vi "DDA.vi"(8 "error in (no error)":errorcluster, 11 "Box Length X (4)":sgl=4.0) -> (0 "error out":errorcluster, 3 "SceneObject out":refnum<vi>)   [LabVIEW 2026, in "XRay CArm.lvclass"]
uses:
  XRay CArm.lvclass
  <vilib>/picture/3D Picture Control/Object/Create Object (drawable).vi
  <vilib>/picture/3D Picture Control/Object/Add Object (reference).vi
  <vilib>/picture/3D Picture Control/NI_3D Picture Control.lvlib
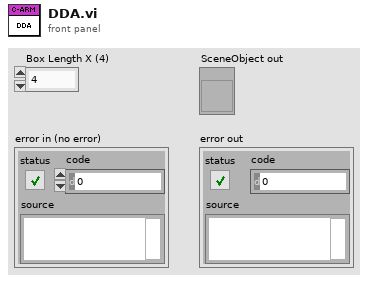
[diagram p1: front panel]
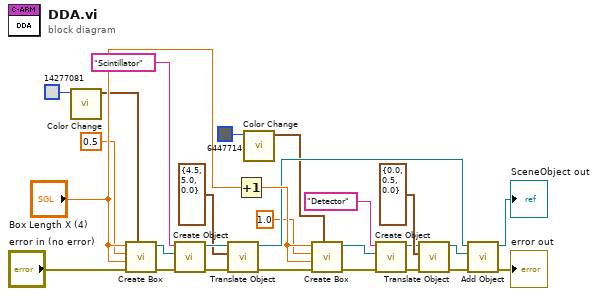
[diagram p0: block diagram]
diagram:
  n1 = call <vilib>:"Color Change.vi"("Color"=u32 14277081) -> ("RGBA"=w14:cluster{"R":sgl, "G":sgl, "B":sgl, "A":sgl})  [unwired: 10 in]
  n2 = call <vilib>:"Create Box.vi"("Color"=w14, "error in (no error)"="error in (no error)", "Length Z"="Box Length X (4)", "Length Y"=sgl 0.5 ("Box Length Y"), "Length X"="Box Length X (4)") -> ("error out"=w13:errorcluster, "New Box Refnum"=w12:refnum<vi>)  [unwired: 5 in]
  n3 = call-poly <vilib>:"Create Object.vi"("error in (no error)"=w13, "Geometry"=w12, "Name"="Scintillator") -> ("error out"=w21:errorcluster, "Scene:New Object"=w11:refnum<vi>)  [unwired: 7 in]
  n4 = call <vilib>:"Translate Object.vi"("error in (no error)"=w21, "Translation"=cluster{"X":sgl, "Y":sgl, "Z":sgl} {"X"=4.5, "Y"=5.0, "Z"=0.0} ("Translation 3"), "Scene.Object In"=w11) -> ("error out"=w23:errorcluster, "Scene.Object Out"=w20:refnum<vi>)  [unwired: 7 in]
  n5 = Increment(x="Box Length X (4)") -> (x+1=w27:sgl)
  n6 = call <vilib>:"Color Change.vi"("Color"=u32 6447714) -> ("RGBA"=w3:cluster{"R":sgl, "G":sgl, "B":sgl, "A":sgl})  [unwired: 10 in]
  n7 = call <vilib>:"Create Box.vi"("Color"=w3, "error in (no error)"=w23, "Length Z"=w27, "Length Y"=sgl 1.0 ("Box Length Y 2"), "Length X"=w27) -> ("error out"=w4:errorcluster, "New Box Refnum"=w5:refnum<vi>)  [unwired: 5 in]
  n8 = call-poly <vilib>:"Create Object.vi"("error in (no error)"=w4, "Geometry"=w5, "Name"="Detector") -> ("error out"=w19:errorcluster, "Scene:New Object"=w6:refnum<vi>)  [unwired: 7 in]
  n9 = call <vilib>:"Translate Object.vi"("error in (no error)"=w19, "Translation"=cluster{"X":sgl, "Y":sgl, "Z":sgl} {"X"=0.0, "Y"=0.5, "Z"=0.0} ("Translation 4"), "Scene.Object In"=w6) -> ("error out"=w24:errorcluster, "Scene.Object Out"=w18:refnum<vi>)  [unwired: 7 in]
  n10 = call-poly <vilib>:"Add Object.vi"("error in (no error)"=w24, "New Object In"=w18, "Scene Object In"=w20) -> ("error out"=→"error out":errorcluster, "Scene Object Out"=→"SceneObject out":refnum<vi>)  [unwired: 6 in, 1 out]
